vi "2.2 Steering Chooser.vi"() -> ()   [LabVIEW 2011]
doc: "TODO: important As of 10/27 this VI only works for the Drive option\n\nWaypoint Monitor takes two things from the global variable - the list of waypoints and\nthe position of the robot at the time.\n\nIt compares the current position to the position of the current waypoint, and if that distance\nis less than the required accuracy the current waypoint value is incremented"
uses:
  2 Typedefs/heading.ctl
  2x3-RIO-OCU Comm/2x3 Typedefs/ocuWaypoint.ctl
  2x3-RIO-OCU Comm/2x3 Typedefs/waypointTypes.ctl
  2 Typedefs/UTM Location.ctl
  2 Typedefs/Velocity.ctl
  2 Globals/2 Global.vi
panel:
  out "Robot\nHeading":T1 format="%05.1f"
  out "Angle to waypt":T1 format="%05.1f"
  out "Distance to Waypoint":T2
  out "Robot UTM Location":T3
  out "Waypoint":T4 {"Point Type" items=["Drive", "Round Port", "Round Starboard", "Stay"]}
  out "desired delta heading":T1 format="%05.1f"
  # "Waypoint Monitor simply turns the rudder to aim the boat towards the next waypoint.\n\nTODO: currently only implements Drive waypoints. Also this is extremely stupid.\nImplement avoidance, stay-in-area, and maybe a PID loop."
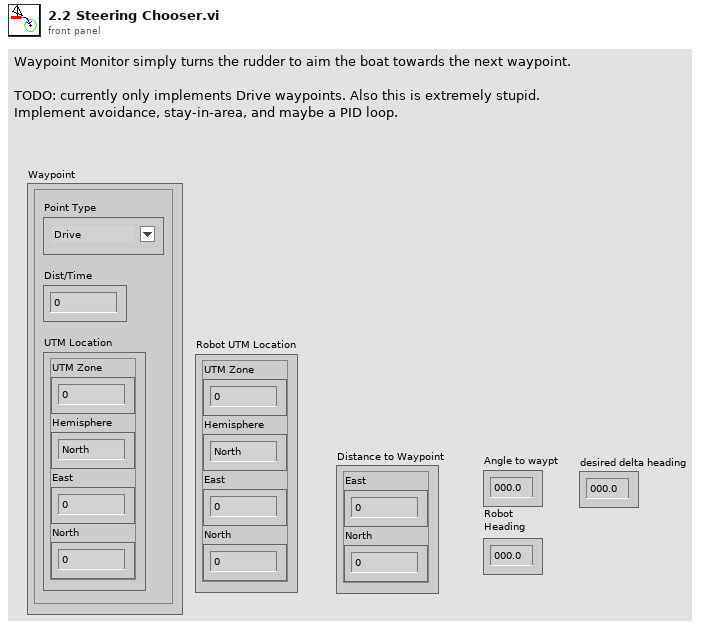
[diagram p1: front panel]
types:
  T1 = typedef "heading.ctl" = dbl
  T2 = typedef "Velocity.ctl" = cluster{"East":dbl, "North":dbl}
  T3 = typedef "UTM Location.ctl" = cluster{"UTM Zone":dbl, "Hemisphere":enum16{"North", "South"}, "East":dbl, "North":dbl}
  T4 = typedef "ocuWaypoint.ctl" = cluster{"Point Type":T5, "Dist/Time":dbl, "UTM Location":T3}
  T5 = typedef "waypointTypes.ctl" = u16
  T6 = typedef "ocuWaypoints.ctl" = cluster{"Waypoints Array":T4[], "Current Waypoint":dbl}
  T7 = cluster{"UTM Zone":dbl, "Hemisphere":u16, "East":dbl, "North":dbl}
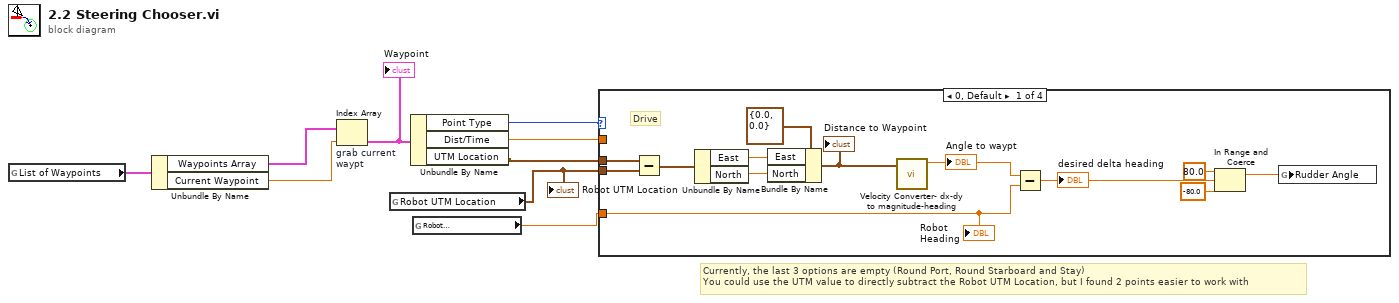
[diagram p0: block diagram]
diagram:
  # "Currently, the last 3 options are empty (Round Port, Round Starboard and Stay)\nYou could use the UTM value to directly subtract the Robot UTM Location, but I found 2 points easier to work with"
  n1 = global read "2 Global.vi" "List of Waypoints"() -> (w7:T6)
  n2 = Unbundle By Name(w7) -> ("Waypoints Array"=w9:T4[], "Current Waypoint"=w8:dbl)
  n3 = Index Array "grab current\nwaypt"(array=w9, index=w8) -> (element=w4:T4)
  "Waypoint" <- w4
  n4 = global read "2 Global.vi" "Robot UTM Location"() -> (w6:T3)
  "Robot UTM Location" <- w6
  n5 = Unbundle By Name(w4) -> ("Point Type"=w1:T5, "Dist/Time"=w2:dbl, "UTM Location"=w3:T3)
  n6 = global read "2 Global.vi" "Robot\nHeading"() -> (w5:T1)
  n7 = case shown="0, Default" w1 {
    tunnel: w3 -> [w22 _ _ _]
    tunnel: w6 -> [w21 _ _ _]
    tunnel: w5 -> [w15 _ _ _]
    tunnel: w2 -> [_ _ _ _]
    frame 0, Default {
      # "Drive"
      n8 = Subtract(x=w22, y=w21) -> (x-y=w20:T7)
      n9 = Unbundle By Name(w20) -> ("East"=w19:dbl, "North"=w18:dbl)
      n10 = Bundle By Name(cluster=T2 {"East"=0.0, "North"=0.0} ("Vector In"), "East"=w19, "North"=w18) -> (w16:T2)
      "Distance to Waypoint" <- w16
      n11 = call "Velocity Converter- dx-dy to magnitude-heading.vi"("Vector In"=w16) -> ("Heading Out"=w10:T1)  [unwired: 9 in, 1 out]
      "Angle to waypt" <- w10
      n12 = Subtract(x=w10, y=w15) -> (x-y=w14:T1)
      "desired delta heading" <- w14
      n13 = In Range and Coerce(upper limit=T1 80.0, x=w14, lower limit=T1 -80.0) -> (coerced(x)=w11:T1)  [unwired: 1 out]
      n14 = global write "2 Global.vi" "Rudder Angle"(w11) -> ()
      "Robot\nHeading" <- w15
    }
    frame 1 {
      # "Round Port"
    }
    frame 2 {
      # "Round Starboard"
    }
    frame 3 {
      # "Stay"
    }
  }
